vi "Lex String.vi"(8 "Error In":errorcluster, 11 "Input":string) -> (0 "Error Out":errorcluster, 3 "Tokens":refnum<class "Abstract.lvclass">[](array[class]))   [LabVIEW 2018, in "Toolkit.lvlib"]
uses:
  Toolkit.lvlib
  Tokens/Abstract/Abstract.lvclass
  Readers/String/String.lvclass
  D:/Users/cfield/Code/Field R&D Services/Mustache/trunk/src/Toolkit/Readers/Abstract/Abstract.lvclass
  Lexer/Lexer.lvclass
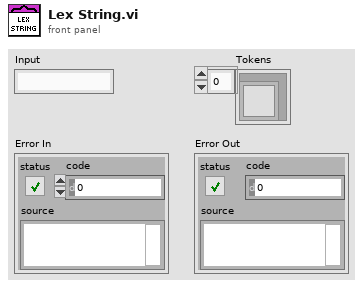
[diagram p1: front panel]
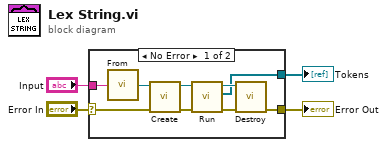
[diagram p0: block diagram]
diagram:
  n1 = case shown="No Error" "Error In" {
    selector: "Error In" -> [w8 w14]
    tunnel: [w9 _] -> w4
    tunnel: [w7 w14] -> w2
    tunnel: "Input" -> [w6 _]
    frame No Error {
      n2 = call "From.vi"("String"=w6) -> ("String"=w5:refnum<class "String.lvclass">)
      n3 = call "Create.vi"("Error In"=w8, "Reader"=w5) -> ("Error Out"=w10:errorcluster, "Parser"=w13:refnum<class "Lexer.lvclass">)  [unwired: 8 in]
      n4 = call "Run.vi"("Error In"=w10, "Parser In"=w13) -> ("Error Out"=w11:errorcluster, "Tokens"=w9:refnum<class "Abstract.lvclass">[], "Parser Out"=w12:refnum<class "Lexer.lvclass">)  [unwired: 7 in]
      n5 = call "Destroy.vi"("Error In"=w11, "Parser"=w12) -> ("Error Out"=w7:errorcluster)  [unwired: 9 in]
    }
    frame Error {
    }
  }
  "Tokens" <- w4
  "Error Out" <- w2
